vi "Generate Large Error.vi"   [LabVIEW 2024]
uses:
  CLI Class/Output.ctl
  CLI Class/CLI.lvclass
types:
  T1 = typedef "CLI.lvclass/Output.ctl" = enum16{"StdOut", "StdErr"}
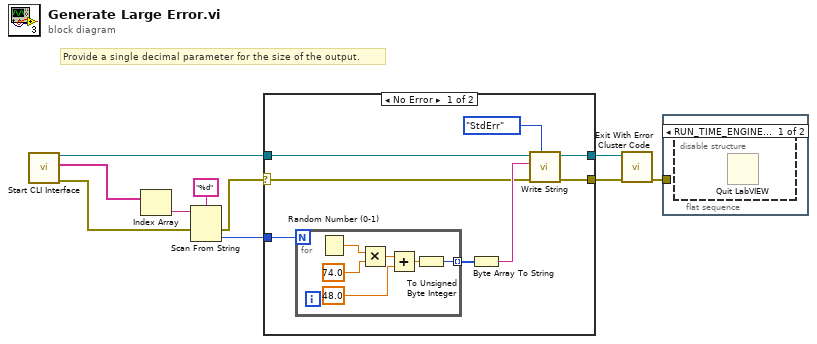
[diagram p0: block diagram]
diagram:
  # "Provide a single decimal parameter for the size of the output."
  n1 = call "Start CLI Interface.vi"() -> ("error out"=w7:errorcluster, "Custom Parameters"=w9:string[], "CLI out"=w2:refnum<class "CLI.lvclass">)  [unwired: 8 in, 1 out]
  n2 = Index Array(array=w9) -> (element=w8:string)  [unwired: 1 in]
  n3 = Scan From String(format string="%d", input string=w8, error in=w7) -> (error out=w1:errorcluster, output 1=w5:i32)  [unwired: 2 in, 2 out]
  n4 = case shown="No Error" w1 {
    selector: w1 -> [w12 w25]
    tunnel: w5 -> [w18 _]
    tunnel: [w16 w25] -> w4
    tunnel: [w15 w26] -> w3
    tunnel: w2 -> [w14 w26]
    frame No Error {
      n5 = for {
        N: w18 -> [_]
        tunnel: [w19] -> w17 mode=indexing
        n6 = Random Number (0-1)() -> (number: 0 to 1=w20:dbl)
        n7 = Multiply(x=w20, y=74.0) -> (x*y=w22:dbl)
        n8 = Add(x=w22, y=48.0) -> (x+y=w24:dbl)
        n9 = To Unsigned Byte Integer(number=w24) -> (unsigned 8bit integer=w19:u8)
      }
      n10 = Byte Array To String(unsigned byte array=w17) -> (string=w13:string)
      n11 = call "Write String.vi"("Output (StdOut)"=Output."StdErr", "error in (no error)"=w12, "Text to Write"=w13, "CLI in"=w14) -> ("error out"=w16:errorcluster, "CLI out"=w15:refnum<class "CLI.lvclass">)  [unwired: 6 in]
    }
    frame Error {
    }
  }
  n12 = call "Exit With Error Cluster Code.vi"("error in (no error)"=w4, "CLI in"=w3) -> ("error out"=w10:errorcluster)  [unwired: 9 in]
  n13 = flat-sequence {
    tunnel: w10 -> [_]
    frame #0 {
      n14 = disable-structure shown="RUN_TIME_ENGINE==True" {
        frame condition #0 {
          n15 = Quit LabVIEW() -> ()  [unwired: 1 in]
        }
        frame condition #1 (active) {
        }
      }
    }
  }
